vi "Tree_GetPath.vi"(6 "i":i32, 9 "level":i32, 10 "# Folders":i32, 11 "Path":path) -> (2 "indent":i32, 3 "path":string)   [LabVIEW 2022 SP3]
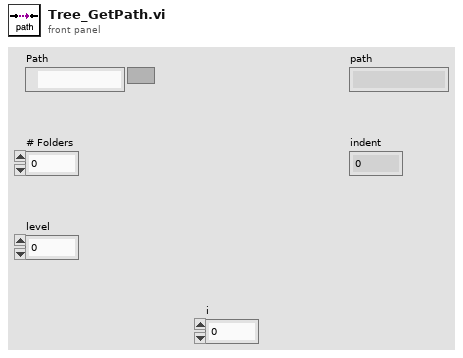
[diagram p1: front panel]
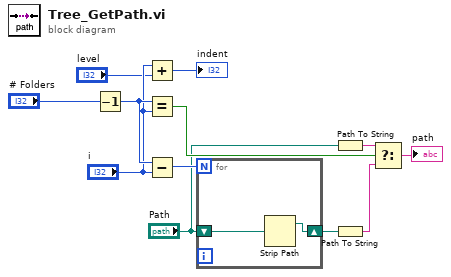
[diagram p0: block diagram]
diagram:
  n1 = Decrement(x="# Folders") -> (x-1=w12:i32)
  n2 = Add(x="i", y="level") -> (x+y=→"indent":i32)
  n3 = Equal?(x=w12, y="i") -> (x = y?=w5:bool)
  n4 = Subtract(x=w12, y="i") -> (x-y=w11:i32)
  n5 = for {
    N: w11 -> [_]
    shift-right: [w14] -> w8
    shift-left: "Path" -> [w13]
    n6 = Strip Path(path=w13) -> (stripped path=w14:path)  [unwired: 1 out]
  }
  n7 = Path To String(path="Path") -> (string=w1:string)
  n8 = Path To String(path=w8) -> (string=w7:string)
  n9 = Select(t=w1, s=w5, f=w7) -> (s? t:f=→"path":string)
